vi "Supports Terminal.vi"(8 "error in (no error)":errorcluster, 11 "SerialResource in":refnum<class "SerialResource.lvclass">) -> (0 "error out":errorcluster, 2 "Supports Terminal":bool, 3 "SerialResource out":refnum<class "SerialResource.lvclass">)   [LabVIEW 2020, in "PicoG-Core.lvlib" / "SerialResource.lvclass"]
doc: "This property determines whether the resource supports the IG Stream Terminal functionality or not. This should generally be true for Resource implementations that wrap an IG Stream implementation and false otherwise. To provide support, a child class must override this property to return a true value and also override the Connection property to supply the stream that can be utilized with the terminal."
uses:
  SerialResource.lvclass
  SerialResource.lvclass/SerialResource.ctl
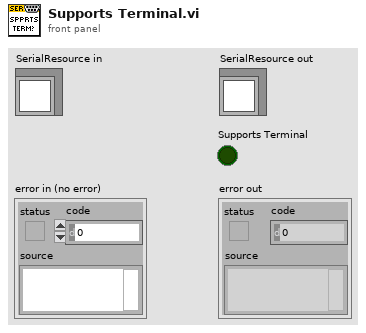
[diagram p1: front panel]
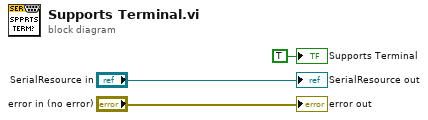
[diagram p0: block diagram]
diagram:
  "error out" <- "error in (no error)"
  "SerialResource out" <- "SerialResource in"
  "Supports Terminal" <- TRUE ("Supports Terminal")
